vi "Brower View Insert Subpanel.vi"(8 "error in (no error)":errorcluster, 11 "Brower View in":refnum<class "Brower View.lvclass">) -> (0 "error out":errorcluster, 3 "Brower View out":refnum<class "Brower View.lvclass">)   [LabVIEW 2015, in "Brower View.lvclass"]
uses:
  Brower View.lvclass
  Brower View.lvclass/Brower View.ctl
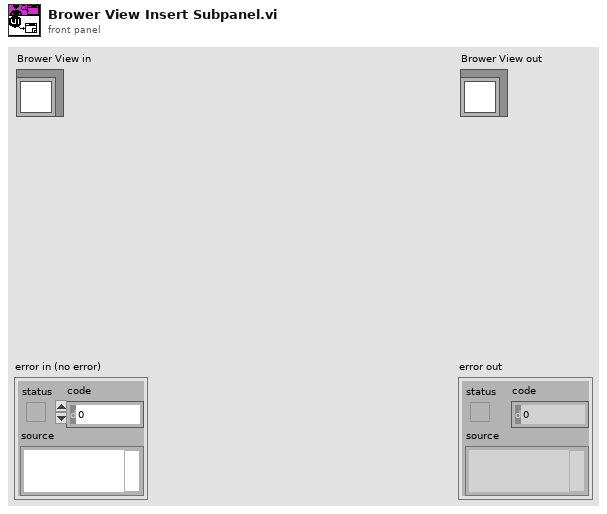
[diagram p1: front panel]
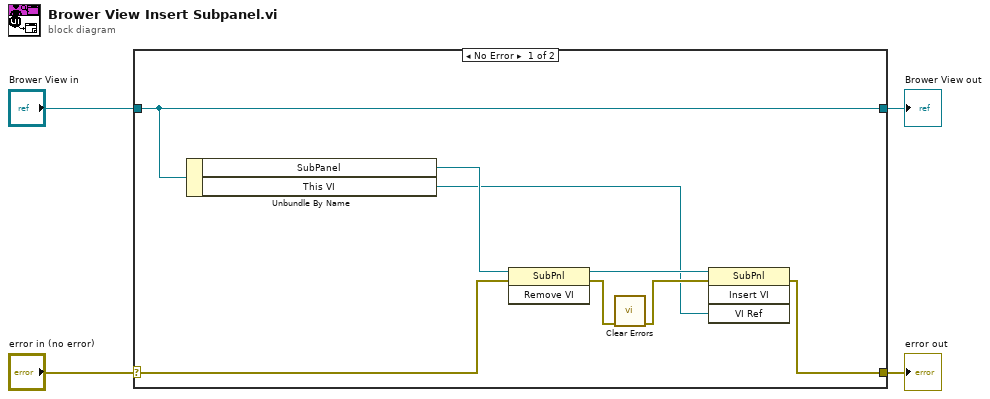
[diagram p0: block diagram]
diagram:
  n1 = case shown="No Error" "error in (no error)" {
    selector: "error in (no error)" -> [w10 w14]
    tunnel: [w5 w14] -> w3
    tunnel: [w12 w13] -> w1
    tunnel: "Brower View in" -> [w12 w13]
    frame No Error {
      n2 = Unbundle By Name(w12) -> ("SubPanel"=w11:refnum<vi>, "This VI"=w6:refnum<vi>)
      n3 = invoke class="SubPnl" method="Remove VI"(reference=w11, error in=w10) -> (reference out=w7:refnum<vi>, error out=w9:errorcluster)  [unwired: 1 in, 1 out]
      n4 = call <vilib>:"Clear Errors.vi"("error in (no error)"=w9) -> ("error out"=w8:errorcluster)  [unwired: 5 in, 1 out]
      n5 = invoke class="SubPnl" method="Insert VI"(reference=w7, error in=w8, "VI Ref"=w6) -> (error out=w5:errorcluster)  [unwired: 1 in, 3 out]
    }
    frame Error {
    }
  }
  "error out" <- w3
  "Brower View out" <- w1
